vi "GetClassName.vi"(0 "reference in":refnum<class "G#Object.lvclass">, 5 "error in (no error)":errorcluster) -> (14 "reference out":refnum<class "G#Object.lvclass">, 15 "class name":string, 16 "lvlib hierarchy":string[](array[string]), 17 "full class name":string, 19 "error out":errorcluster)   [LabVIEW 2017, in "G#Object.lvclass"]
doc: "Returns the class name, full class name , lvlib hierarchy for the specified object."
uses:
  G#Object.lvclass
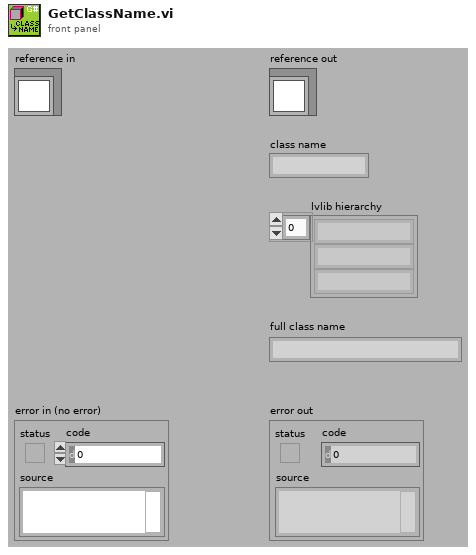
[diagram p1: front panel]
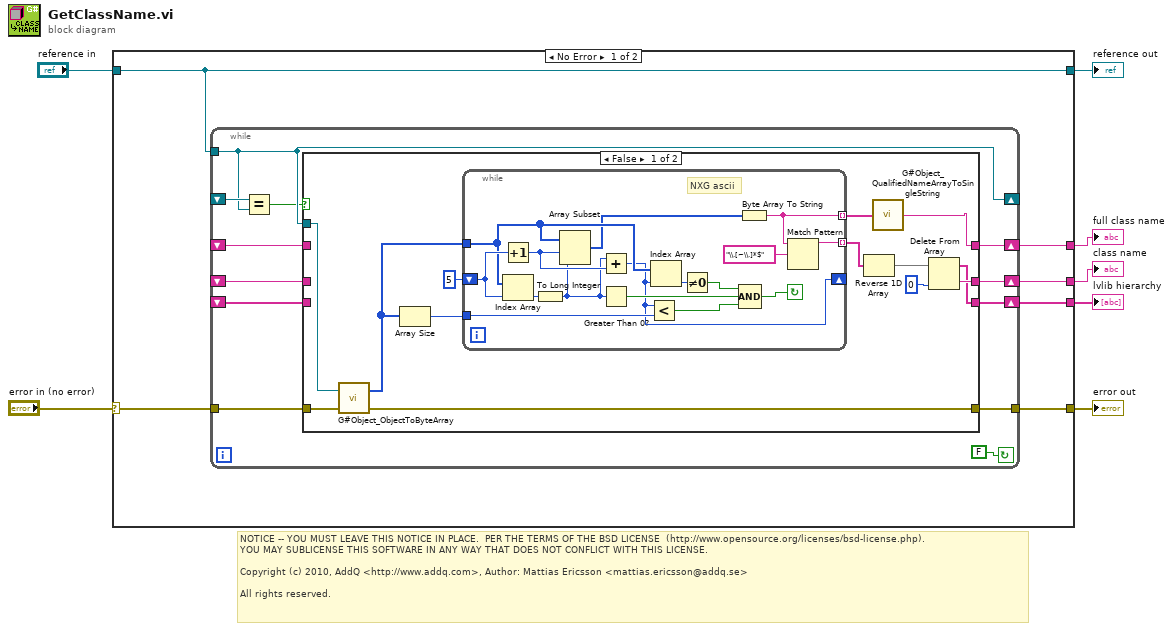
[diagram p0: block diagram]
diagram:
  # "NOTICE -- YOU MUST LEAVE THIS NOTICE IN PLACE.  PER THE TERMS OF THE BSD LICENSE  (http://www.opensource.org/licenses/bsd-license.php).\nYOU MAY SUBLICENSE THIS SOFTWARE IN ANY WAY THAT DOES NOT CONFLICT WITH THIS LICENSE.\n\nCopyright (c) 2010, AddQ <http://www.addq.com>, Author: Mattias Ericsson <mattias.ericsson@addq.se>\n\nAll rights reserved."
  n1 = case shown="No Error" "error in (no error)" {
    selector: "error in (no error)" -> [w13 w60]
    tunnel: "reference in" -> [w8 w59]
    tunnel: [w11 w60] -> w3
    tunnel: [w10 _] -> w7
    tunnel: [w9 _] -> w6
    tunnel: [w12 _] -> w5
    tunnel: [w8 w59] -> w2
    frame No Error {
      n2 = while {
        tunnel: [w25] -> w11
        tunnel: w13 -> [w24]
        tunnel: w8 -> [w18]
        shift-right: [w18] -> _
        shift-left: _ -> [w19]
        shift-right: [w21] -> w10
        shift-left: _ -> [w17]
        shift-right: [w22] -> w9
        shift-left: _ -> [w16]
        shift-right: [w23] -> w12
        shift-left: _ -> [w15]
        stop <- FALSE continue-if-true
        n3 = Equal?(x=w19, y=w18) -> (x = y?=w14:bool)
        n4 = case shown="False" w14 {
          tunnel: [w28 w56] -> w25
          tunnel: w24 -> [w29 w56]
          tunnel: [w26 w55] -> w23
          tunnel: [w35 w57] -> w22
          tunnel: [w34 w58] -> w21
          tunnel: w18 -> [w31 _]
          tunnel: w17 -> [_ w58]
          tunnel: w16 -> [_ w57]
          tunnel: w15 -> [_ w55]
          frame False {
            n5 = call "G#Object_ObjectToByteArray.vi"("reference"=w31, "error in (no error)"=w29) -> ("unsigned byte array"=w30:u8[], "error out"=w28:errorcluster)  [unwired: 16 in]
            n6 = Array Size(array=w30) -> (size(s)=w32:i32)
            n7 = while {
              shift-right: [w43] -> _
              shift-left: 5 -> [w49]
              tunnel: w32 -> [w52]
              tunnel: [w50] -> w33 mode=indexing
              tunnel: [w45] -> w27 mode=indexing
              tunnel: w30 -> [w46]
              stop <- w41 continue-if-true
              # "NXG ascii"
              n8 = Increment(x=w49) -> (x+1=w44:i32)
              n9 = Index Array(array=w46, index=w49) -> (element=w40:u8)
              n10 = To Long Integer(number=w40) -> (32bit integer=w39:i32)
              n11 = Array Subset(array=w46, index=w44, length=w39) -> (w42:u8[])
              n12 = Add(x=w39, y=w44) -> (x+y=w43:i32)
              n13 = Greater Than 0?(x=w39) -> (x > 0?=w54:bool)
              n14 = Less?(x=w43, y=w52) -> (x < y?=w53:bool)
              n15 = Index Array(array=w46, index=w43) -> (element=w48:u8)
              n16 = Not Equal To 0?(x=w48) -> (x != 0?=w47:bool)
              n17 = Byte Array To String(unsigned byte array=w42) -> (string=w45:string)
              n18 = Compound Arithmetic op=AND(w47, w54, w53) -> (w41:bool)
              n19 = Match Pattern(string=w45, regular expression="\\.[~\\.]*$") -> (before substring=w50:string)  [unwired: 4 out]
            }
            n20 = Reverse 1D Array(array=w33) -> (reversed array=w36:string[])
            n21 = call "G#Object_QualifiedNameArrayToSingleString.vi"("Fully Qualified Array"=w27) -> ("Fully Qualified String"=w26:string)
            n22 = Delete From Array(array=w36, index=0) -> (deleted portion=w35:string, array with subset deleted=w34:string[])  [unwired: 1 in]
          }
          frame True {
          }
        }
      }
    }
    frame Error {
    }
  }
  "reference out" <- w2
  "class name" <- w6
  "lvlib hierarchy" <- w7
  "full class name" <- w5
  "error out" <- w3
